vi "UI Panels - Create.vi"(8 "error in (no error)":errorcluster, 11 "Panels_XControl":refnum<vi>) -> (0 "error out":errorcluster, 3 "Panels_XControl":refnum<vi>)   [LabVIEW 2013, in "UI Panels.lvlib"]
uses:
  UI Panels.lvlib
  Panels_XControl.xctl
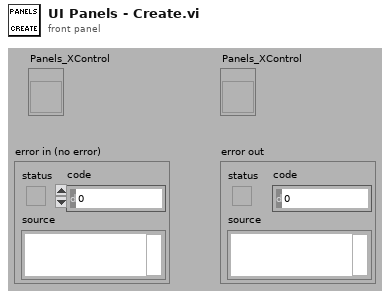
[diagram p1: front panel]
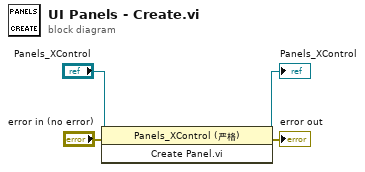
[diagram p0: block diagram]
diagram:
  n1 = invoke on="Invoke Node" class="Panels_XControl (严格)" method="Create Panel.vi"(reference="Panels_XControl", error in="error in (no error)") -> (reference out=→"Panels_XControl":refnum<vi>, error out=→"error out":errorcluster)  [unwired: 1 in, 1 out]
